vi "UPCONVERSION.vi"() -> ()   [LabVIEW 2011]
uses:
  <vilib>/Utility/file.llb/Write To Spreadsheet File (DBL).vi
panel:
  out "No of Scan":i32
  in  "Stop Taking Data":bool
  in  "UP CONVERSION":T1(tab)
  in  "Final File Path":path
  in  "Current File Path":string="C:\\Users\\nshukla\\Desktop\\2\\"
  in  "Position (units)":dbl
  in  "Velocity value (units/s) in":dbl
  out "Current position (units)":dbl
  out "Velocity value (units/s) out":dbl
  in  "Start Data Accusition":bool
  out "Position Time Zero":dbl
  out "GRAPH":T2(graph)
  out "XY Graph":cluster{"Y":dbl[], "Y":dbl[]}[](graph)
  out "Final Graph":cluster{"Y":dbl[], "Y":dbl[]}[](graph)
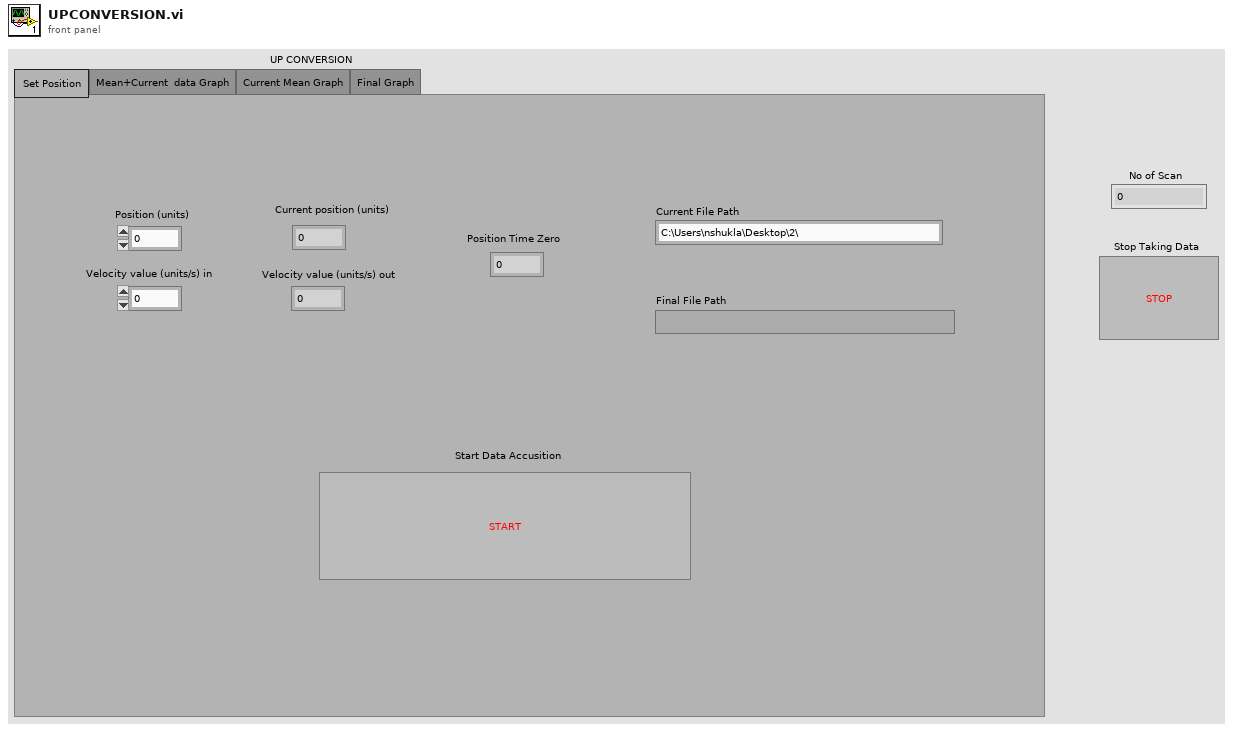
[diagram p1: front panel]
types:
  T1 = enum32{"Set Position ", "Mean+Current  data Graph", "Current Mean Graph", "Final Graph"}
  T2 = cluster{"XY Graph ":cluster{"Y":dbl[], "Y":dbl[]}[], "XY Graph":cluster{"Y":dbl[], "Y":dbl[]}[]}
  T3 = enum16{"open", "replace", "create", "open or create", "replace or create", "replace or create with confirmation"}
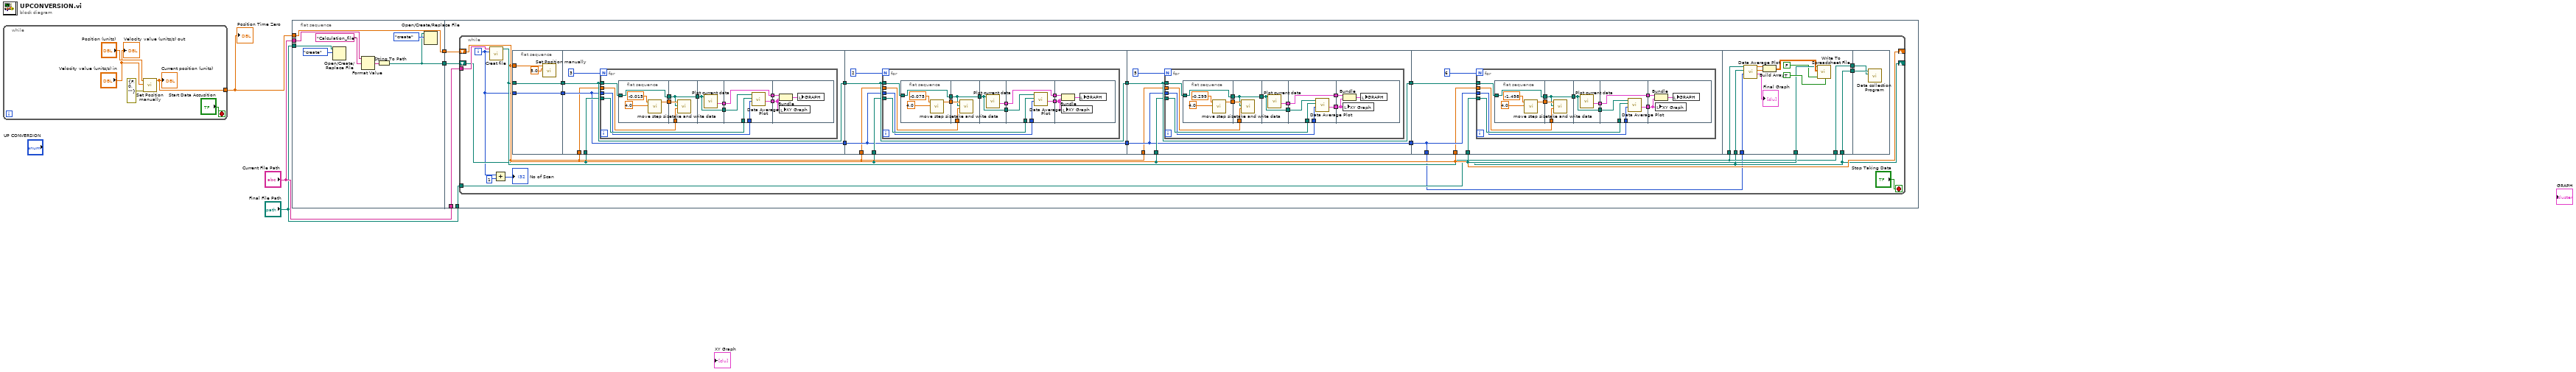
[diagram p0: block diagram]
diagram:
  n1 = while {
    tunnel: [w8] -> w5
    stop <- "Start Data Accusition" stop-if-true
    n2 = call "Set Position manually.vi"("error in (no error)"=errorcluster {"status"=FALSE, "code"=0, "source"=""}, "Velocity value (units/s) in"="Velocity value (units/s) in", "Displacement (units)"="Position (units)") -> ("Current position (units)"=w8:dbl)  [unwired: 7 in, 1 out]
    "Current position (units)" <- w8
    "Velocity value (units/s) out" <- "Velocity value (units/s) in"
  }
  "Position Time Zero" <- w5
  n3 = flat-sequence {
    tunnel: w5 -> [w18]
    tunnel: [w18] -> w4
    tunnel: [w13] -> w3
    tunnel: "Final File Path" -> [w17]
    tunnel: "Current File Path" -> [w12]
    tunnel: "Final File Path" -> [w19]
    tunnel: "Current File Path" -> [w20]
    tunnel: w3 -> [w21]
    tunnel: w4 -> [w22]
    frame #0 {
      n4 = Open/Create/Replace File(file path (use dialog)=w17, operation (0:open)=T3."create") -> ()  [unwired: 4 in, 3 out]
      n5 = Format Value(string ("")=w12, format string="Calculation_file") -> (output string=w14:string)  [unwired: 1 in]
      n6 = String To Path(string=w14) -> (path=w13:path)
      n7 = Open/Create/Replace File(file path (use dialog)=w13, operation (0:open)=T3."create") -> ()  [unwired: 4 in, 3 out]
    }
    frame #1 {
      n8 = while {
        shift-right: [w33] -> _
        shift-left: w22 -> [w33]
        shift-right: [w29] -> _
        shift-left: w21 -> [w29]
        tunnel: w20 -> [w32]
        tunnel: w19 -> [w31]
        i -> [w27]
        stop <- "Stop Taking Data" stop-if-true
        n9 = call "Creat file.vi"("Numeric"=w27, "File Path"=w32) -> ("Path"=w30:path)  [unwired: 9 in]
        n10 = Add(x=w27, y=1) -> (x+y=→"No of Scan":i32)
        n11 = flat-sequence {
          tunnel: w33 -> [w46]
          tunnel: [w44] -> w42
          tunnel: w30 -> [w44]
          tunnel: w27 -> [w43]
          tunnel: [w43] -> w37
          tunnel: w42 -> [w50]
          tunnel: [w50] -> w41
          tunnel: w29 -> [w49]
          tunnel: w37 -> [w48]
          tunnel: [w48] -> w36
          tunnel: w33 -> [w47]
          tunnel: w41 -> [w83]
          tunnel: [w83] -> w39
          tunnel: w29 -> [w82]
          tunnel: w36 -> [w81]
          tunnel: [w81] -> w35
          tunnel: w33 -> [w80]
          tunnel: [w117] -> w40
          tunnel: w39 -> [w117]
          tunnel: w29 -> [w116]
          tunnel: w35 -> [w115]
          tunnel: [w115] -> w34
          tunnel: w33 -> [w114]
          tunnel: w40 -> [w150]
          tunnel: w29 -> [w149]
          tunnel: w34 -> [w147]
          tunnel: [w147] -> w28
          tunnel: w33 -> [w146]
          tunnel: w31 -> [w185]
          tunnel: w30 -> [w184]
          tunnel: w29 -> [w183]
          tunnel: w28 -> [w182]
          tunnel: w30 -> [w179]
          tunnel: w29 -> [w180]
          tunnel: [w180] -> w24
          tunnel: [w179] -> w23
          tunnel: w24 -> [w192]
          tunnel: w23 -> [w191]
          frame #0 {
            n12 = call "Set Position manually.vi"("Velocity value (units/s) in"=5.0 ("Velocity for detecting position zero"), "Displacement (units)"=w46) -> ()  [unwired: 8 in, 2 out]
          }
          frame #1 {
            n13 = for {
              N: 3 ("Set count 1") -> [_]
              tunnel: w50 -> [w62]
              tunnel: w49 -> [w58]
              tunnel: w48 -> [w55]
              tunnel: w47 -> [w54]
              n14 = flat-sequence {
                tunnel: [w64] -> w53
                tunnel: [w63] -> w52
                tunnel: w62 -> [w63]
                tunnel: [w68] -> w61
                tunnel: w54 -> [w67]
                tunnel: w52 -> [w68]
                tunnel: w53 -> [w69]
                tunnel: w61 -> [w70]
                tunnel: [w71] -> w60
                tunnel: [w70] -> w57
                tunnel: w60 -> [w76]
                tunnel: [w76] -> w59
                tunnel: w58 -> [w75]
                tunnel: w57 -> [w74]
                tunnel: [w73] -> w56
                tunnel: w55 -> [w72]
                tunnel: w59 -> [w78]
                tunnel: w56 -> [w77]
                frame #0 {
                  n15 = call "move step size.vi"("Velocity value (units/s) in"=4.0 ("Velocity 1"), "Displacement (units)"=-0.015 ("Step Size 1")) -> ("Current position (units)"=w64:dbl)  [unwired: 8 in, 1 out]
                }
                frame #1 {
                  n16 = call "take and write data.vi"("y"=w67, "Path"=w68, "Current position (units)"=w69) -> ()  [unwired: 9 in]
                }
                frame #2 {
                  n17 = call "Plot current data.vi"("file path (dialog if empty)"=w70) -> ("XY Graph"=w71:cluster{"Y":dbl[], "Y":dbl[]}[])  [unwired: 8 in]
                }
                frame #3 {
                  n18 = call "Data Average Plot.vi"("No of element"=w72, "Average file path"=w75, "Current file path"=w74) -> ("XY Graph"=w73:cluster{"Y":dbl[], "Y":dbl[]}[])  [unwired: 4 in, 2 out]
                }
                frame #4 {
                  n19 = Bundle("XY Graph"=w78, "XY Graph"=w77) -> (w79:T2)  [unwired: 1 in]
                  n20 = local write "XY Graph"(w77) -> ()
                  n21 = local write "GRAPH"(w79) -> ()
                }
              }
            }
          }
          frame #2 {
            n22 = for {
              N: 2 ("Set count 2") -> [_]
              tunnel: w83 -> [w95]
              tunnel: w82 -> [w91]
              tunnel: w81 -> [w88]
              tunnel: w80 -> [w87]
              n23 = flat-sequence {
                tunnel: [w97] -> w86
                tunnel: [w96] -> w85
                tunnel: w95 -> [w96]
                tunnel: [w101] -> w94
                tunnel: w87 -> [w100]
                tunnel: w85 -> [w101]
                tunnel: w86 -> [w102]
                tunnel: w94 -> [w103]
                tunnel: [w104] -> w93
                tunnel: [w103] -> w90
                tunnel: w93 -> [w109]
                tunnel: [w109] -> w92
                tunnel: w91 -> [w108]
                tunnel: w90 -> [w107]
                tunnel: [w106] -> w89
                tunnel: w88 -> [w105]
                tunnel: w92 -> [w111]
                tunnel: w89 -> [w110]
                frame #0 {
                  n24 = call "move step size.vi"("Velocity value (units/s) in"=4.0 ("Velocity 2"), "Displacement (units)"=-0.075 ("Step Size 2")) -> ("Current position (units)"=w97:dbl)  [unwired: 8 in, 1 out]
                }
                frame #1 {
                  n25 = call "take and write data.vi"("y"=w100, "Path"=w101, "Current position (units)"=w102) -> ()  [unwired: 9 in]
                }
                frame #2 {
                  n26 = call "Plot current data.vi"("file path (dialog if empty)"=w103) -> ("XY Graph"=w104:cluster{"Y":dbl[], "Y":dbl[]}[])  [unwired: 8 in]
                }
                frame #3 {
                  n27 = call "Data Average Plot.vi"("No of element"=w105, "Average file path"=w108, "Current file path"=w107) -> ("XY Graph"=w106:cluster{"Y":dbl[], "Y":dbl[]}[])  [unwired: 4 in, 2 out]
                }
                frame #4 {
                  n28 = Bundle("XY Graph"=w111, "XY Graph"=w110) -> (w112:T2)  [unwired: 1 in]
                  n29 = local write "XY Graph"(w110) -> ()
                  n30 = local write "GRAPH"(w112) -> ()
                }
              }
            }
          }
          frame #3 {
            n31 = for {
              N: 5 ("Set count 3") -> [_]
              tunnel: w117 -> [w128]
              tunnel: w116 -> [w124]
              tunnel: w115 -> [w121]
              tunnel: w114 -> [w120]
              n32 = flat-sequence {
                tunnel: [w130] -> w119
                tunnel: [w129] -> w118
                tunnel: w128 -> [w129]
                tunnel: [w134] -> w127
                tunnel: w120 -> [w133]
                tunnel: w118 -> [w134]
                tunnel: w119 -> [w135]
                tunnel: w127 -> [w136]
                tunnel: [w137] -> w126
                tunnel: [w136] -> w123
                tunnel: w126 -> [w142]
                tunnel: [w142] -> w125
                tunnel: w124 -> [w141]
                tunnel: w123 -> [w140]
                tunnel: [w139] -> w122
                tunnel: w121 -> [w138]
                tunnel: w125 -> [w144]
                tunnel: w122 -> [w143]
                frame #0 {
                  n33 = call "move step size.vi"("Velocity value (units/s) in"=4.0 ("Velocity 3"), "Displacement (units)"=-0.299 ("Step Size 3")) -> ("Current position (units)"=w130:dbl)  [unwired: 8 in, 1 out]
                }
                frame #1 {
                  n34 = call "take and write data.vi"("y"=w133, "Path"=w134, "Current position (units)"=w135) -> ()  [unwired: 9 in]
                }
                frame #2 {
                  n35 = call "Plot current data.vi"("file path (dialog if empty)"=w136) -> ("XY Graph"=w137:cluster{"Y":dbl[], "Y":dbl[]}[])  [unwired: 8 in]
                }
                frame #3 {
                  n36 = call "Data Average Plot.vi"("No of element"=w138, "Average file path"=w141, "Current file path"=w140) -> ("XY Graph"=w139:cluster{"Y":dbl[], "Y":dbl[]}[])  [unwired: 4 in, 2 out]
                }
                frame #4 {
                  n37 = Bundle("XY Graph"=w144, "XY Graph"=w143) -> (w145:T2)  [unwired: 1 in]
                  n38 = local write "XY Graph"(w143) -> ()
                  n39 = local write "GRAPH"(w145) -> ()
                }
              }
            }
          }
          frame #4 {
            n40 = for {
              N: 6 -> [_]
              tunnel: w150 -> [w161]
              tunnel: w149 -> [w157]
              tunnel: w147 -> [w154]
              tunnel: w146 -> [w153]
              n41 = flat-sequence {
                tunnel: [w163] -> w152
                tunnel: [w162] -> w151
                tunnel: w161 -> [w162]
                tunnel: [w167] -> w160
                tunnel: w153 -> [w166]
                tunnel: w151 -> [w167]
                tunnel: w152 -> [w168]
                tunnel: w160 -> [w169]
                tunnel: [w170] -> w159
                tunnel: [w169] -> w156
                tunnel: w159 -> [w175]
                tunnel: [w175] -> w158
                tunnel: w157 -> [w174]
                tunnel: w156 -> [w173]
                tunnel: [w172] -> w155
                tunnel: w154 -> [w171]
                tunnel: w158 -> [w177]
                tunnel: w155 -> [w176]
                frame #0 {
                  n42 = call "move step size.vi"("Velocity value (units/s) in"=4.0 ("Velocity 4"), "Displacement (units)"=-1.498 ("Step Size 4")) -> ("Current position (units)"=w163:dbl)  [unwired: 8 in, 1 out]
                }
                frame #1 {
                  n43 = call "take and write data.vi"("y"=w166, "Path"=w167, "Current position (units)"=w168) -> ()  [unwired: 9 in]
                }
                frame #2 {
                  n44 = call "Plot current data.vi"("file path (dialog if empty)"=w169) -> ("XY Graph"=w170:cluster{"Y":dbl[], "Y":dbl[]}[])  [unwired: 8 in]
                }
                frame #3 {
                  n45 = call "Data Average Plot.vi"("No of element"=w171, "Average file path"=w174, "Current file path"=w173) -> ("XY Graph"=w172:cluster{"Y":dbl[], "Y":dbl[]}[])  [unwired: 4 in, 2 out]
                }
                frame #4 {
                  n46 = Bundle("XY Graph"=w177, "XY Graph"=w176) -> (w178:T2)  [unwired: 1 in]
                  n47 = local write "XY Graph"(w176) -> ()
                  n48 = local write "GRAPH"(w178) -> ()
                }
              }
            }
          }
          frame #5 {
            n49 = call "Data Average Plot.vi"("No of element"=w182, "Average file path"=w183, "Current file path"=w184) -> ("XY Graph"=→"Final Graph":cluster{"Y":dbl[], "Y":dbl[]}[], "Y Out"=w188:dbl[], "X Out"=w187:dbl[])  [unwired: 4 in]
            n50 = Build Array(w187, w188) -> (w189:dbl[][])
            n51 = call-poly <vilib>:"Write To Spreadsheet File.vi"("transpose? (no:F)"=TRUE, "append to file? (new file:F)"=FALSE, "2D data"=w189, "file path (dialog if empty)"=w185) -> ()  [unwired: 4 in, 1 out]
          }
          frame #6 {
            n52 = call "Data collection Program.vi"("Current File Name"=w191, "Average file path"=w192) -> ()  [unwired: 9 in, 1 out]
          }
        }
      }
    }
  }
